vi "SiosIfmSearchUSBDevices.vi"() -> (0 "Array":cluster{string, i16}[](array[cluster]), 1 "Number of SIOS USB Devices":i32)   [LabVIEW 2009]
uses:
  siosifm.dll
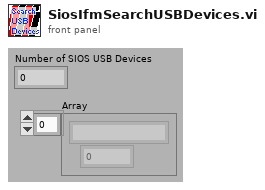
[diagram p1: front panel]
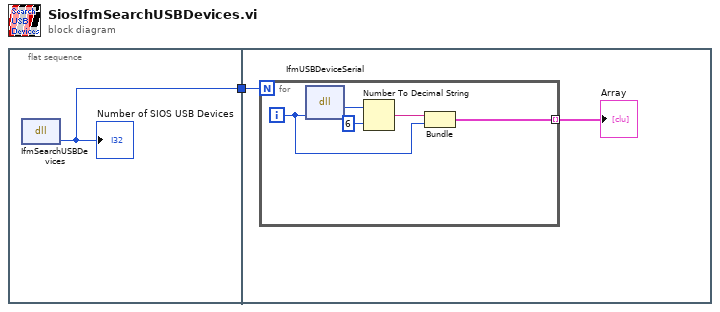
[diagram p0: block diagram]
diagram:
  n1 = flat-sequence {
    tunnel: [w2] -> w1
    tunnel: w1 -> [w3]
    frame #0 {
      n2 = dll-call lib="D:/Support/Labview/RE-10/SIOS_IfmDLL/siosifm.dll" fn="IfmSearchUSBDevices"() -> (w2:i32)  [unwired: 3 in, 2 out]
      "Number of SIOS USB Devices" <- w2
    }
    frame #1 {
      n3 = for {
        N: w3 -> [_]
        tunnel: [w7] -> w4 mode=indexing
        i -> [w6]
        n4 = dll-call lib="D:/Support/Labview/RE-10/SIOS_IfmDLL/siosifm.dll" fn="IfmUSBDeviceSerial"("uiniqeId"=w6) -> (w8:i32)  [unwired: 4 in, 2 out]
        n5 = Number To Decimal String(number=w8, width (-)=i16 6 ("Breite (-)")) -> (decimal integer string=w9:string)
        n6 = Bundle(w9, w6) -> (w7:cluster{string, i32})  [unwired: 1 in]
      }
      "Array" <- w4
    }
  }
